vi "row3.vi"(11 "Array in":i32[](array[numeric])) -> (2 "Array out":i32[](array[numeric]), 3 "Enum":T1(ring))   [LabVIEW 2016]
uses:
  <vilib>/NXT/Block Support/NXT_OutputPort.ctl
  <vilib>/NXT/Block Support/NXT_InputPort.ctl
  <vilib>/NXT/Subs/ColorSensorColors.ctl
  <vilib>/NXT/NXTIO Xnodes/NXTIONodeSubVIs/NXTStopMotors.vi
  <vilib>/NXT/NXTIO Xnodes/NXTIONodeSubVIs/NXTMotorRunDistance.vi
  <vilib>/NXT/NXTIO Xnodes/NXTIONodeSubVIs/LEGOMotorStatus.vi
  <vilib>/NXT/NXTIO Xnodes/NXTIONodeSubVIs/NXTMoveMotors.vi
  <vilib>/NXT/NXTIO Xnodes/NXTIONodeSubVIs/LEGOResetMotors.vi
  <vilib>/NXT/Subs/LVHSConnector.ctl
  <vilib>/NXT/NXTIO Xnodes/AddressXNode/NXTIOAddress.xnode
  <vilib>/NXT/NXTIO Xnodes/NXTIOXNode/NXTIO.xnode
  <vilib>/NXT/LegoClasses/BrickReference/BrickReference.lvclass
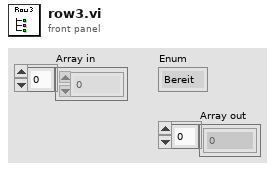
[diagram p1: front panel]
types:
  T1 = enum16{"Bereit", "Move 1", "Reference_pos", "Wait", "row1_check", "row2_check", "row3_check", "return", "move2", "move3", "move4", "move5", "end"}
  T2 = enum16{"forward", "pause1", "right1", "pause2", "right2", "pause3", "end"}
  T3 = typedef "NXT_OutputPort.ctl" = u8
  T4 = typedef "ColorSensorColors.ctl" = enum16{"No Color", "Black", "Blue", "Green", "Yellow", "Red", "White", "Brown"}
  T5 = cluster{"Output Port":T3, "Output Port 2":T3, "Output Port 3":T3}
  T6 = typedef "LVHSConnector.ctl" = refnum<class "BrickReference.lvclass">
  T7 = typedef "NXT_InputPort.ctl" = u32
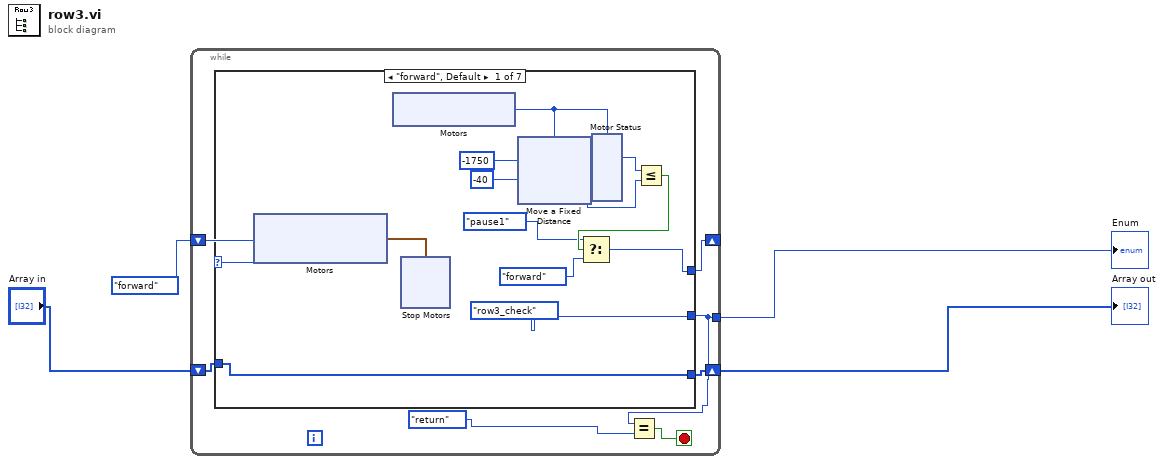
[diagram p0: block diagram]
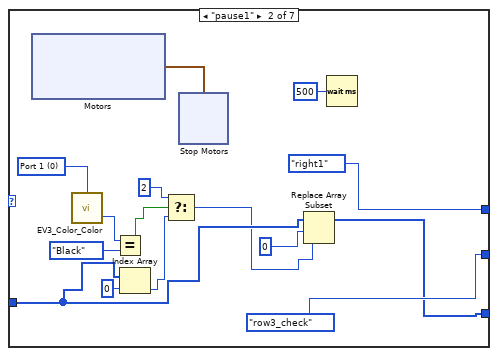
[diagram p2: hidden frame]
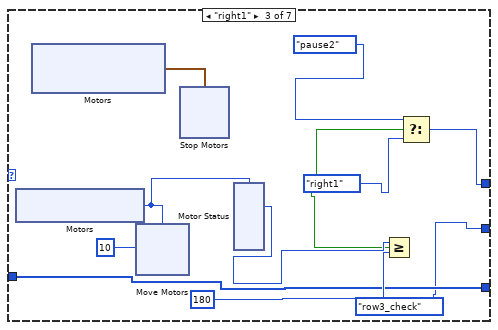
[diagram p3: hidden frame]
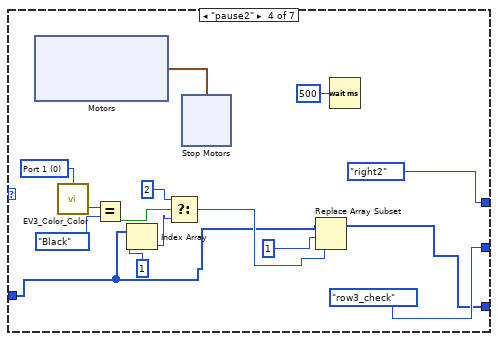
[diagram p4: hidden frame]
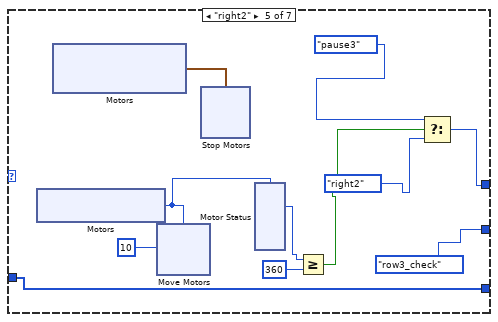
[diagram p5: hidden frame]
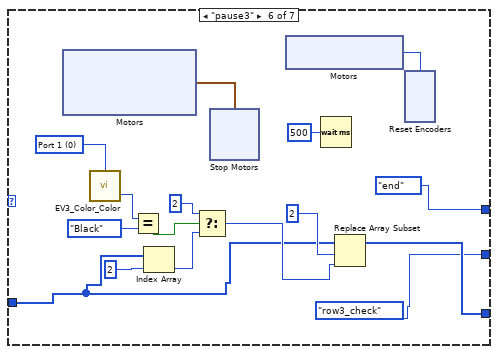
[diagram p6: hidden frame]
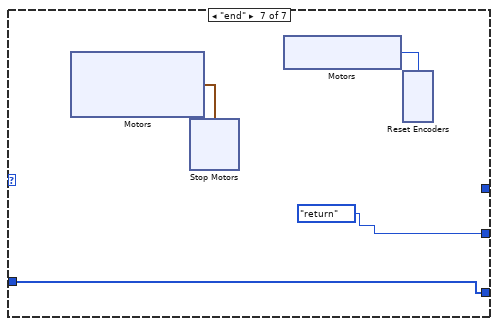
[diagram p7: hidden frame]
diagram:
  n1 = while {
    shift-right: [w9] -> _
    shift-left: T2."forward" -> [w10]
    tunnel: [w8] -> w2
    shift-right: [w6] -> w4
    shift-left: "Array in" -> [w7]
    stop <- w11 stop-if-true
    n2 = case shown="\"forward\", Default" w10 {
      tunnel: [w12 T2."right1" w72 T2."right2" w128 T2."end" _] -> w9
      tunnel: [T1."row3_check" T1."row3_check" T1."row3_check" T1."row3_check" T1."row3_check" T1."row3_check" T1."return"] -> w8
      tunnel: [w22 w49 w71 w106 w125 w163 w186] -> w6
      tunnel: w7 -> [w22 w52 w71 w104 w125 w160 w186]
      frame "forward", Default {
        w18 = -1750 ("Distance 1")
        n3 = xnode "Motors"() -> ("Motor"=w23:cluster{"Port":T3, "Port":T3})
        n4 = xnode "Motors"() -> ("Motor"=w17:T3)
        n5 = xnode "Stop Motors"("Motors"=w23) -> ()  [unwired: 1 in, 1 out]
        n6 = xnode "Move a Fixed Distance"("Speed 1"=i8 -40, "Distance 1"=w18, "Motors"=w17) -> ("NXT/EV3"=w16:T6)  [unwired: 1 in]
        n7 = xnode "Motor Status"("Motors"=w17, "NXT/EV3"=w16) -> ("Position 1"=w19:i32)  [unwired: 2 out]
        n8 = Less Or Equal?(x=w19, y=w18) -> (x <= y?=w15:bool)
        n9 = Select(t=T2."pause1", s=w15, f=T2."forward") -> (s? t:f=w12:T2)
      }
      frame "pause1" {
        w62 = T7 0 items=["Port 1", "Port 2", "Port 3", "Port 4"] ("Port (Port 1)")
        n10 = xnode "Motors"() -> ("Motor"=w63:cluster{"Port":T3, "Port":T3, "Port":T3})
        n11 = call <vilib>:"EV3_Color_Color.vi"("Port (Port 1)"=w62) -> ("Detected Color"=w61:T4)  [unwired: 2 in, 1 out]
        n12 = Equal?(x=w61, y=ColorSensorColors."Black") -> (x = y?=w58:bool)
        n13 = Index Array(array=w52, index=0 ("disabled index (col)")) -> (element=w53:i32)
        n14 = Select(t=2 ("disabled index (col)"), s=w58, f=w53) -> (s? t:f=w50:i32)
        n15 = xnode "Stop Motors"("Motors"=w63) -> ()  [unwired: 1 in, 1 out]
        n16 = Replace Array Subset(array=w52, new element=w50, index=0 ("disabled index (col)")) -> (w49:i32[])
        n17 = Wait (ms)(milliseconds to wait=u32 500) -> ()  [unwired: 1 out]
      }
      frame "right1" {
        n18 = xnode "Motors"() -> ("Motor"=w79:T3)
        n19 = xnode "Motors"() -> ("Motor"=w78:cluster{"Port":T3, "Port":T3})
        n20 = xnode "Move Motors"("Power/Speed 1"=i8 10, "Motors"=w79) -> ()  [unwired: 1 in, 1 out]
        n21 = xnode "Stop Motors"("Motors"=w78) -> ()  [unwired: 1 in, 1 out]
        n22 = xnode "Motor Status"("Motors"=w79) -> ("Position 1"=w77:i32)  [unwired: 1 in, 2 out]
        n23 = Greater Or Equal?(x=w77, y=180) -> (x >= y?=w75:bool)
        n24 = Select(t=T2."pause2", s=w75, f=T2."right1") -> (s? t:f=w72:T2)
      }
      frame "pause2" {
        w116 = T7 0 items=["Port 1", "Port 2", "Port 3", "Port 4"] ("Port (Port 1)")
        n25 = xnode "Motors"() -> ("Motor"=w117:cluster{"Port":T3, "Port":T3, "Port":T3})
        n26 = call <vilib>:"EV3_Color_Color.vi"("Port (Port 1)"=w116) -> ("Detected Color"=w115:T4)  [unwired: 2 in, 1 out]
        n27 = Equal?(x=w115, y=ColorSensorColors."Black") -> (x = y?=w112:bool)
        n28 = Index Array(array=w104, index=1 ("disabled index (col)")) -> (element=w103:i32)
        n29 = Select(t=2 ("disabled index (col)"), s=w112, f=w103) -> (s? t:f=w107:i32)
        n30 = xnode "Stop Motors"("Motors"=w117) -> ()  [unwired: 1 in, 1 out]
        n31 = Replace Array Subset(array=w104, new element=w107, index=1 ("disabled index (col)")) -> (w106:i32[])
        n32 = Wait (ms)(milliseconds to wait=u32 500) -> ()  [unwired: 1 out]
      }
      frame "right2" {
        n33 = xnode "Motors"() -> ("Motor"=w133:T3)
        n34 = xnode "Motors"() -> ("Motor"=w132:cluster{"Port":T3, "Port":T3})
        n35 = xnode "Move Motors"("Power/Speed 1"=i8 10, "Motors"=w133) -> ()  [unwired: 1 in, 1 out]
        n36 = xnode "Stop Motors"("Motors"=w132) -> ()  [unwired: 1 in, 1 out]
        n37 = xnode "Motor Status"("Motors"=w133) -> ("Position 1"=w127:i32)  [unwired: 1 in, 2 out]
        n38 = Greater Or Equal?(x=w127, y=360) -> (x >= y?=w131:bool)
        n39 = Select(t=T2."pause3", s=w131, f=T2."right2") -> (s? t:f=w128:T2)
      }
      frame "pause3" {
        w171 = T7 0 items=["Port 1", "Port 2", "Port 3", "Port 4"] ("Port (Port 1)")
        n40 = xnode "Motors"() -> ("Motor"=w172:cluster{"Port":T3, "Port":T3, "Port":T3})
        n41 = call <vilib>:"EV3_Color_Color.vi"("Port (Port 1)"=w171) -> ("Detected Color"=w170:T4)  [unwired: 2 in, 1 out]
        n42 = Equal?(x=w170, y=ColorSensorColors."Black") -> (x = y?=w168:bool)
        n43 = Index Array(array=w160, index=2 ("disabled index (row)")) -> (element=w159:i32)
        n44 = Select(t=2 ("disabled index (col)"), s=w168, f=w159) -> (s? t:f=w165:i32)
        n45 = xnode "Stop Motors"("Motors"=w172) -> ()  [unwired: 1 in, 1 out]
        n46 = xnode "Motors"() -> ("Motor"=w158:T3)
        n47 = Wait (ms)(milliseconds to wait=u32 500) -> ()  [unwired: 1 out]
        n48 = Replace Array Subset(array=w160, new element=w165, index=2 ("index (row)")) -> (w163:i32[])
        n49 = xnode "Reset Encoders"("Motors"=w158) -> ()  [unwired: 1 in, 1 out]
      }
      frame "end" {
        n50 = xnode "Motors"() -> ("Motor"=w187:cluster{"Port":T3, "Port":T3, "Port":T3})
        n51 = xnode "Stop Motors"("Motors"=w187) -> ()  [unwired: 1 in, 1 out]
        n52 = xnode "Motors"() -> ("Motor"=w184:T3)
        n53 = xnode "Reset Encoders"("Motors"=w184) -> ()  [unwired: 1 in, 1 out]
      }
    }
    n54 = Equal?(x=w8, y=T1."return") -> (x = y?=w11:bool)
  }
  "Array out" <- w4
  "Enum" <- w2
